vi "Launch Target Actor.vi"() -> (0 "error out":errorcluster)   [LabVIEW 2024]
uses:
  Devices/DAQmx/AO/AO DAQmx DC CFG/AO DAQmx DC CFG.lvclass
  Devices/DAQmx/Thermo/Thermometer DAQmx RTD Cont CFG/Thermometer DAQmx RTD Cont CFG.lvclass
  Devices/DAQmx/AI/AI Current DAQmx Cont CFG/AI Current DAQmx Cont CFG.lvclass
  Devices/DAQmx/AI/AI Voltage DAQmx Cont CFG/AI Voltage DAQmx Cont CFG.lvclass
  Virtual Instruments/PA Remote on Const Channel with DBL Strategy/Perform Action Remote on Const Channel with DBL Strategy.lvclass
  Virtual Instruments/PA Remote on Const Channel with 3DBL Strategy/Perform Action Remote on Const Channel with 3DBL Strategy.lvclass
  Virtual Instruments/PA Remote on Const Channel with 2DBL Strategy/Perform Action Remote on Const Channel with 2DBL Strategy.lvclass
  MSS Target Actor/MSS Target Actor/MSS Target Actor.lvclass/MSS Target Actor.ctl
  <vilib>/ni/Actors/Network Endpoint Actors/Protocols/Network Stream Strategy/Netowrk Stream Listener/Network Stream Listener.lvclass
  <vilib>/ActorFramework/Actor/Actor.lvclass
  MSS Target Actor/MSS Target Actor/MSS Target Actor.lvclass
  C:/Program Files/National Instruments/LabVIEW 2024/vi.lib/ni/Actors/Network Endpoint Actors/Protocols/Network Stream Strategy/Network Stream/Network Stream.lvclass
  C:/Program Files/National Instruments/LabVIEW 2024/vi.lib/ni/Actors/Network Endpoint Actors/Abstract Classes/Message Stream/Message Stream.lvclass
  C:/Program Files/National Instruments/LabVIEW 2024/vi.lib/ni/Actors/Network Endpoint Actors/Protocols/Network Stream Strategy/Netowrk Stream Listener/Network Stream Listener.lvclass
  C:/Program Files/National Instruments/LabVIEW 2024/vi.lib/ActorFramework/Actor/Actor.lvclass
  D:/git/HAL/HAL/MSS Target Actor/MSS Target Actor/MSS Target Actor.lvclass
  D:/git/HAL/HAL/MSS Target Actor/IMSS Target Actor/IMSS Target Actor.lvclass
  C:/Program Files/National Instruments/LabVIEW 2024/vi.lib/ni/Actors/Network Endpoint Actors/Nested Endpoint Caller/Nested Endpoint Caller/Nested Endpoint Caller.lvclass
panel:
  # "Target"
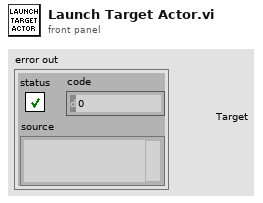
[diagram p1: front panel]
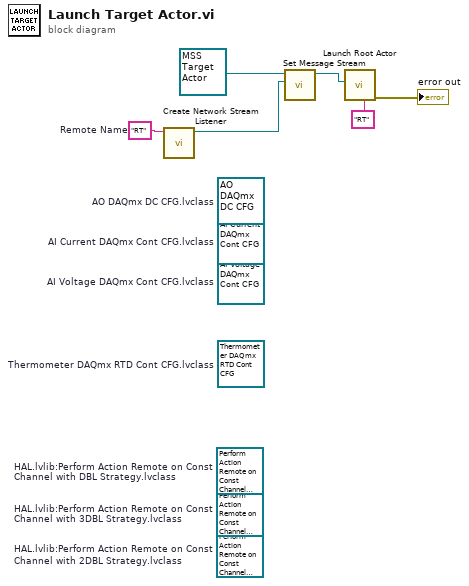
[diagram p0: block diagram]
diagram:
  (unwired) refnum<class "Perform Action Remote on Const Channel with 2DBL Strategy.lvclass"> refnum  # HAL.lvlib:Perform Action Remote on Const Channel with 2DBL Strategy.lvclass
  (unwired) refnum<class "Perform Action Remote on Const Channel with 3DBL Strategy.lvclass"> refnum  # HAL.lvlib:Perform Action Remote on Const Channel with 3DBL Strategy.lvclass
  (unwired) refnum<class "Perform Action Remote on Const Channel with DBL Strategy.lvclass"> refnum  # HAL.lvlib:Perform Action Remote on Const Channel with DBL Strategy.lvclass
  (unwired) refnum<class "AI Voltage DAQmx Cont CFG.lvclass"> refnum  # AI Voltage DAQmx Cont CFG.lvclass
  (unwired) refnum<class "AI Current DAQmx Cont CFG.lvclass"> refnum  # AI Current DAQmx Cont CFG.lvclass
  (unwired) refnum<class "Thermometer DAQmx RTD Cont CFG.lvclass"> refnum  # Thermometer DAQmx RTD Cont CFG.lvclass
  (unwired) refnum<class "AO DAQmx DC CFG.lvclass"> refnum  # AO DAQmx DC CFG.lvclass
  w6 = "RT"  # Remote Name
  n1 = call <vilib>:"Create Network Stream Listener.vi"("Name"=w6) -> ("Network Stream Listener"=w1:refnum<class "Network Stream Listener.lvclass">)  [unwired: 10 in]
  n2 = call "Set Message Stream.vi"("Message Stream.lvclass"=w1, "CRIO MSS Test Actor in"=refnum<class "MSS Target Actor.lvclass"> refnum ("MSS Target Actor.lvlib:MSS Target Actor.lvclass")) -> ("CRIO MSS Test Actor out"=w5:refnum<class "MSS Target Actor.lvclass">)  [unwired: 9 in]
  n3 = call <vilib>:"Launch Root Actor.vi"("Debug Alias"="RT", "Actor"=w5) -> ("error out"=→"error out":errorcluster)  [unwired: 8 in, 1 out]
